vi "ExpFitHandle.vi"(8 "error in (no error)":errorcluster, 11 "Stand in":refnum<class "Stand.lvclass">) -> (0 "error out":errorcluster, 3 "Stand out":refnum<class "Stand.lvclass">)   [LabVIEW 2019, in "Stand.lvclass"]
uses:
  Stand.lvclass
  D:/GIT H4000/H4000/src/Device_class/Device.lvclass
  Stand.lvclass/Stand.ctl
  FPGA/TypeDef/DO index.ctl
  FPGA/TypeDef/AI index.ctl
  AI_class/AI.lvclass/AI.ctl
  AnalogComparator_class/AnalogComparator.lvclass/AnalogComparator.ctl
  OscillationClass/OscillationDetector.lvclass/OscillationDetector.ctl
  Device_class/Device.lvclass/Device.ctl
  249e4558-2c97-4a7e-83c2-ea0cef2754e0.vi
  AnalogComparator_class/GetStatus.vi
  OscillationClass/Read DATA.vi
  FPGA_API_class/FPGA API.lvclass
  ExpFitter/ExpFitter.lvclass
  Device_class/Device.lvclass
  AI_class/AI.lvclass
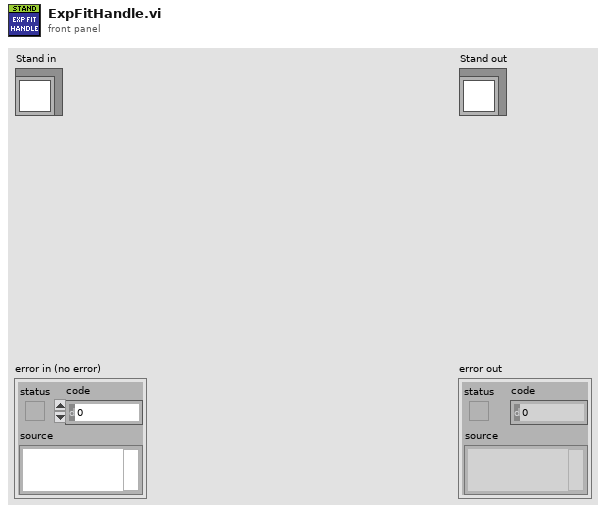
[diagram p1: front panel]
types:
  T1 = typedef "Step_Name.ctl" = enum16{"IDLE", "Filling", "Low Pressure", "Hi Pressure", "Abrupt Pressure Release", "Smooth Pressure Release", "Measuring Leakage Sensor 41.3", "Measuring Leakage Burette 42", "Alarm", "Stop Pump"}
  T2 = typedef "AI index.ctl" = u8
  T3 = typedef "DO index.ctl" = u8
  T4 = typedef "AI_Data.ctl" = cluster{"Stat Data":T5, "OutOfRangeMax":bool, "OutOfRangeMin":bool, "HIHI":bool, "HI":bool, "LO":bool, "LOLO":bool, "DATA N":T6, "DATA PERIOD":T6, "UPPER TH":dbl, "LOWER TH":dbl}
  T5 = typedef "AI Statistics Data.ctl" = cluster{"raw mean":dbl, "scl mean":dbl, "raw mean 1Hz":dbl, "scl mean 1Hz":dbl}
  T6 = typedef "DATA Oscill.ctl" = cluster{"SUM":dbl, "COUNTER":dbl, "MAX CURR":dbl, "MIN CURR":dbl, "AVR":dbl, "MAX":dbl, "MIN":dbl, "DELTA AVR":dbl, "DELTA MAX":dbl, "DELTA MIN":dbl, "PERIOD":dbl}
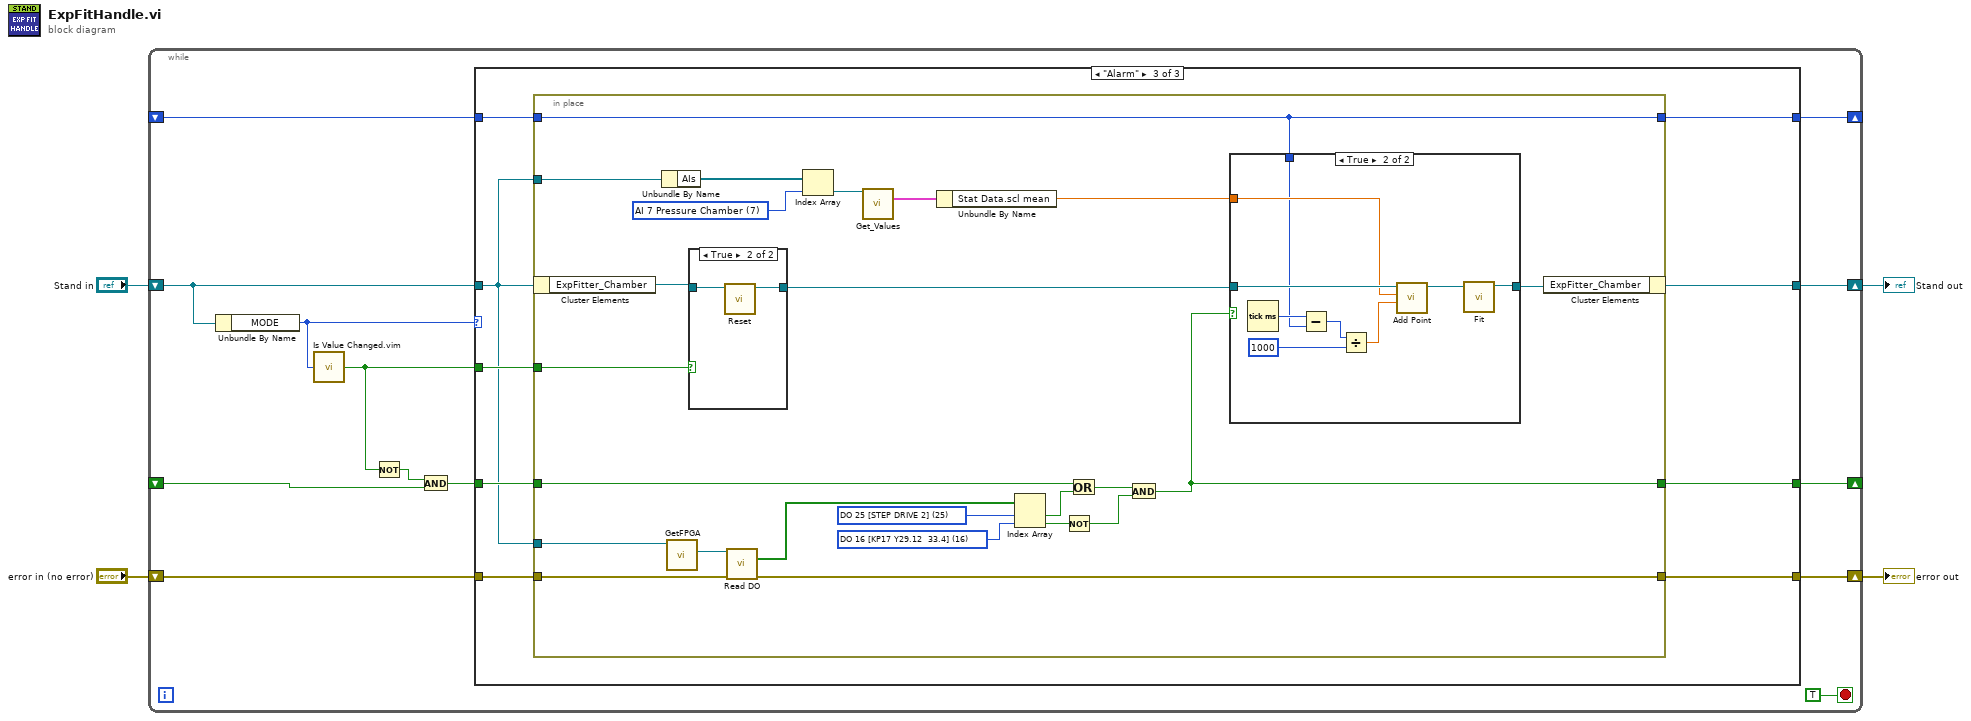
[diagram p0: block diagram]
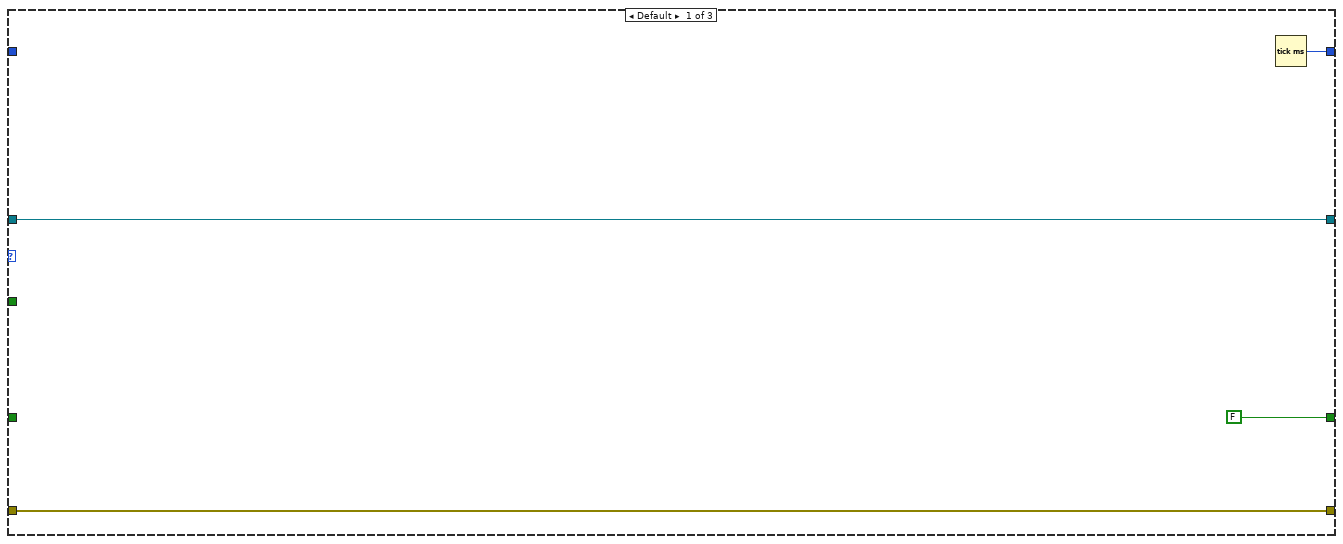
[diagram p2: hidden frame]
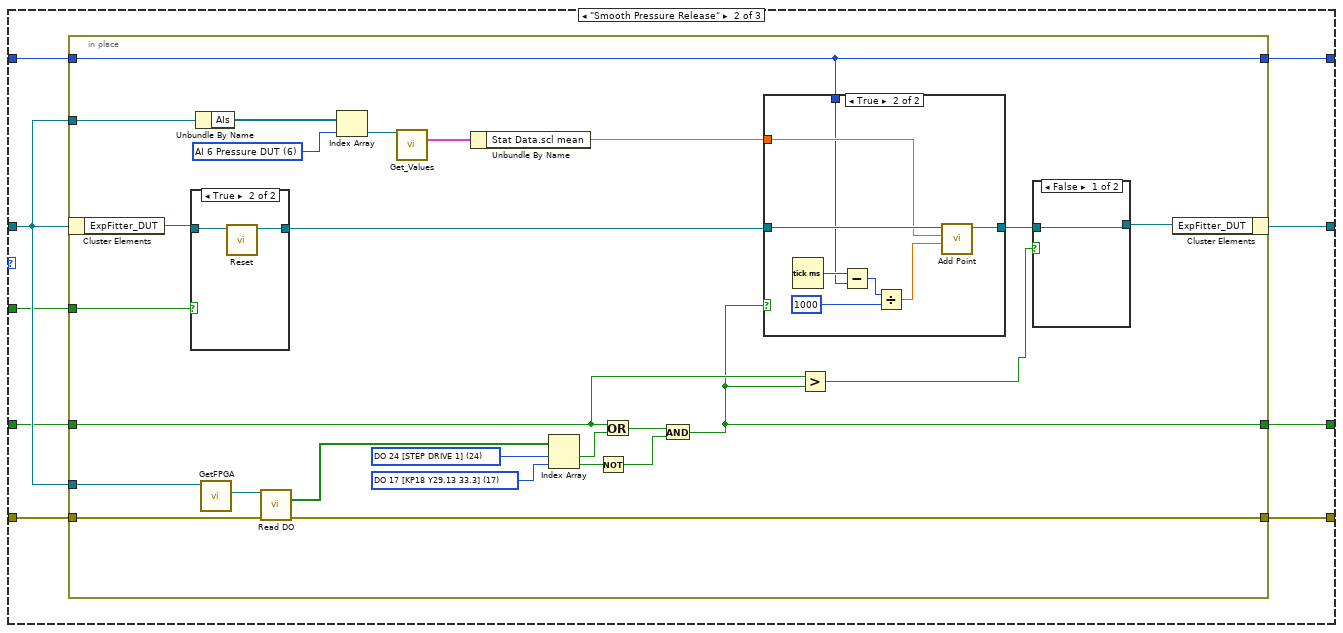
[diagram p3: hidden frame]
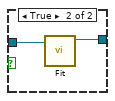
[diagram p4: hidden frame]
diagram:
  n1 = while {
    shift-right: [w15] -> w2
    shift-left: "error in (no error)" -> [w16]
    shift-right: [w17] -> w4
    shift-left: "Stand in" -> [w11]
    shift-right: [w12] -> _
    shift-left: _ -> [w8]
    shift-right: [w10] -> _
    shift-left: _ -> [w9]
    stop <- TRUE stop-if-true
    n2 = Unbundle By Name(w11) -> ("MODE"=w14:T1)
    n3 = call "Is Value Changed.vim"("value"=w14) -> ("changed or first call?"=w5:bool)
    n4 = Not(x=w5) -> (.not. x?=w6:bool)
    n5 = And(x=w6, y=w8) -> (x .and. y?=w7:bool)
    n6 = case shown="\"Alarm\"" w14 {
      tunnel: w11 -> [w21 w24 w72]
      tunnel: [w21 w25 w73] -> w17
      tunnel: w16 -> [w20 w30 w80]
      tunnel: [w20 w26 w74] -> w15
      tunnel: w5 -> [_ w23 w79]
      tunnel: [FALSE w29 w77] -> w12
      tunnel: w7 -> [_ w22 w78]
      tunnel: [w19 w28 w76] -> w10
      tunnel: w9 -> [_ w27 w75]
      frame Default {
        n7 = Tick Count (ms)() -> (millisecond timer value=w19:u32)
      }
      frame "Smooth Pressure Release" {
        n8 = in-place {
          in-place-border: w30 -> [w38]
          in-place-border: w23 -> [w55]
          in-place-border: w24 -> [w53]
          in-place-border: w22 -> [w33]
          in-place-border: [w32] -> w29
          in-place-border: [w39] -> w28
          in-place-border: w27 -> [w39]
          in-place-border: [w37] -> w26
          in-place-border: w24 -> [w36]
          w44 = T2 6 items=["AI 0 Cooling Station Level", "AI 1 Cooling Station Temp", "AI 2 Oil Supply Level", "AI 3 Oil Supply Temp", "AI 4 ", "AI 5 Pressure Haskel", "AI 6 Pressure DUT", "AI 7 Pressure Chamber", "AI 8 Pressure Air inlet", "AI 9 Pressure Air outlet", "AI 10 Pressure Messure Line"] ("AI index")
          w52 = T3 17 items=["DO 0 [KP1] [M12]", "DO 1 [ON KP2] [M21]", "DO 2 [ON KP3] [M24]", "DO 3 [WATER Y18.1 [DO3]]", "DO 4 [WATER Y18.2 [DO4]]", "DO 5 [KP6 Y29.1 33.7]", "DO 6 [KP7 Y29.2 33.8]", "DO 7 [KP8 Y29.3 33.9]", "DO 8 [KP9 Y29.4  33.12]", "DO 9 [KP10 Y29.5 33.1]", "DO 10 [KP11 Y29.6 33.2]", "DO 11 [KP12 Y29.7  33.13]", "DO 12 [KP13 Y29.8  33.11]", "DO 13 [KP14 Y29.9 33.10]", "DO 14 [KP15 Y29.10  33.6]", "DO 15 [KP16 Y29.11  33.5]", "DO 16 [KP17 Y29.12  33.4]", "DO 17 [KP18 Y29.13 33.3]", "DO 18 [AIR KP19]", "DO 19 [STEP DRIVE EN KP20]", "DO 20 [KP21 Y44.1 OPEN]", "DO 21 [ KP22 Y44.1 CLOSE]", "DO 22 [ KP23 Y44.2 OPEN]", "DO 23", "DO 24 [STEP DRIVE 1]", "DO 25 [STEP DRIVE 2]"] ("DO index")
          w51 = T3 24 items=["DO 0 [KP1] [M12]", "DO 1 [ON KP2] [M21]", "DO 2 [ON KP3] [M24]", "DO 3 [WATER Y18.1 [DO3]]", "DO 4 [WATER Y18.2 [DO4]]", "DO 5 [KP6 Y29.1 33.7]", "DO 6 [KP7 Y29.2 33.8]", "DO 7 [KP8 Y29.3 33.9]", "DO 8 [KP9 Y29.4  33.12]", "DO 9 [KP10 Y29.5 33.1]", "DO 10 [KP11 Y29.6 33.2]", "DO 11 [KP12 Y29.7  33.13]", "DO 12 [KP13 Y29.8  33.11]", "DO 13 [KP14 Y29.9 33.10]", "DO 14 [KP15 Y29.10  33.6]", "DO 15 [KP16 Y29.11  33.5]", "DO 16 [KP17 Y29.12  33.4]", "DO 17 [KP18 Y29.13 33.3]", "DO 18 [AIR KP19]", "DO 19 [STEP DRIVE EN KP20]", "DO 20 [KP21 Y44.1 OPEN]", "DO 21 [ KP22 Y44.1 CLOSE]", "DO 22 [ KP23 Y44.2 OPEN]", "DO 23", "DO 24 [STEP DRIVE 1]", "DO 25 [STEP DRIVE 2]"] ("DO index")
          n9 = in-place-cluster #1(w24) -> ("ExpFitter_DUT"=w56:refnum<class "ExpFitter.lvclass">)
          n10 = case shown="True" w55 {
            tunnel: w56 -> [w60 w62]
            tunnel: [w60 w61] -> w54
            frame False {
            }
            frame True {
              n11 = call "Reset.vi"("ExpFitter in"=w62) -> ("ExpFitter out"=w61:refnum<class "ExpFitter.lvclass">)  [unwired: 10 in]
            }
          }
          n12 = Unbundle By Name(w36) -> ("AIs"=w41:refnum<class "AI.lvclass">[])
          n13 = call "GetFPGA.vi"("Device in"=w53) -> ("FPGA API.lvclass"=w50:refnum<class "FPGA API.lvclass">)  [unwired: 10 in]
          n14 = call-dynamic "Read DO.vi"("FPGA API in"=w50, "error in (no error)"=w38) -> ("Ds"=w49:bool[], "error out"=w37:errorcluster)  [unwired: 11 in, 1 out]
          n15 = Index Array(array=w41, index=w44) -> (element=w42:refnum<class "AI.lvclass">)
          n16 = call "Get_Values.vi"("reference in"=w42) -> ("Data"=w43:T4)  [unwired: 14 in]
          n17 = Unbundle By Name(w43) -> ("Stat Data.scl mean"=w40:dbl)
          n18 = Index Array(array=w49, index #1=w51, index #2=w52) -> (element #1=w48:bool, element #2=w46:bool)
          n19 = Not(x=w46) -> (.not. x?=w45:bool)
          n20 = Or(x=w33, y=w48) -> (x .or. y?=w47:bool)
          n21 = And(x=w47, y=w45) -> (x .and. y?=w32:bool)
          n22 = case shown="True" w32 {
            tunnel: w54 -> [w63 w71]
            tunnel: [w63 w64] -> w35
            tunnel: w40 -> [_ w70]
            tunnel: w39 -> [_ w68]
            frame False {
            }
            frame True {
              n23 = Tick Count (ms)() -> (millisecond timer value=w69:u32)
              n24 = Subtract(x=w69, y=w68) -> (x-y=w67:u32)
              n25 = Divide(x=w67, y=u32 1000) -> (x/y=w65:dbl)
              n26 = call "Add Point.vi"("X"=w65, "Y"=w70, "ExpFitter in"=w71) -> ("ExpFitter out"=w64:refnum<class "ExpFitter.lvclass">)  [unwired: 8 in]
            }
          }
          n27 = Greater?(x=w33, y=w32) -> (0:w31:bool)
          n28 = case shown="False" w31 {
            tunnel: w35 -> [w57 w59]
            tunnel: [w57 w58] -> w34
            frame False {
            }
            frame True {
              n29 = call "Fit.vi"("ExpFitter in"=w59) -> ("ExpFitter out"=w58:refnum<class "ExpFitter.lvclass">)  [unwired: 10 in]
            }
          }
          n30 = in-place-cluster #1("ExpFitter_DUT"=w34) -> (w25:refnum<class "Stand.lvclass">)
        }
      }
      frame "Alarm" {
        n31 = in-place {
          in-place-border: w80 -> [w83]
          in-place-border: w79 -> [w103]
          in-place-border: w72 -> [w101]
          in-place-border: w78 -> [w96]
          in-place-border: [w91] -> w77
          in-place-border: [w84] -> w76
          in-place-border: w75 -> [w84]
          in-place-border: [w82] -> w74
          in-place-border: w72 -> [w81]
          w89 = T2 7 items=["AI 0 Cooling Station Level", "AI 1 Cooling Station Temp", "AI 2 Oil Supply Level", "AI 3 Oil Supply Temp", "AI 4 ", "AI 5 Pressure Haskel", "AI 6 Pressure DUT", "AI 7 Pressure Chamber", "AI 8 Pressure Air inlet", "AI 9 Pressure Air outlet", "AI 10 Pressure Messure Line"] ("AI index")
          w100 = T3 16 items=["DO 0 [KP1] [M12]", "DO 1 [ON KP2] [M21]", "DO 2 [ON KP3] [M24]", "DO 3 [WATER Y18.1 [DO3]]", "DO 4 [WATER Y18.2 [DO4]]", "DO 5 [KP6 Y29.1 33.7]", "DO 6 [KP7 Y29.2 33.8]", "DO 7 [KP8 Y29.3 33.9]", "DO 8 [KP9 Y29.4  33.12]", "DO 9 [KP10 Y29.5 33.1]", "DO 10 [KP11 Y29.6 33.2]", "DO 11 [KP12 Y29.7  33.13]", "DO 12 [KP13 Y29.8  33.11]", "DO 13 [KP14 Y29.9 33.10]", "DO 14 [KP15 Y29.10  33.6]", "DO 15 [KP16 Y29.11  33.5]", "DO 16 [KP17 Y29.12  33.4]", "DO 17 [KP18 Y29.13 33.3]", "DO 18 [AIR KP19]", "DO 19 [STEP DRIVE EN KP20]", "DO 20 [KP21 Y44.1 OPEN]", "DO 21 [ KP22 Y44.1 CLOSE]", "DO 22 [ KP23 Y44.2 OPEN]", "DO 23", "DO 24 [STEP DRIVE 1]", "DO 25 [STEP DRIVE 2]"] ("DO index")
          w99 = T3 25 items=["DO 0 [KP1] [M12]", "DO 1 [ON KP2] [M21]", "DO 2 [ON KP3] [M24]", "DO 3 [WATER Y18.1 [DO3]]", "DO 4 [WATER Y18.2 [DO4]]", "DO 5 [KP6 Y29.1 33.7]", "DO 6 [KP7 Y29.2 33.8]", "DO 7 [KP8 Y29.3 33.9]", "DO 8 [KP9 Y29.4  33.12]", "DO 9 [KP10 Y29.5 33.1]", "DO 10 [KP11 Y29.6 33.2]", "DO 11 [KP12 Y29.7  33.13]", "DO 12 [KP13 Y29.8  33.11]", "DO 13 [KP14 Y29.9 33.10]", "DO 14 [KP15 Y29.10  33.6]", "DO 15 [KP16 Y29.11  33.5]", "DO 16 [KP17 Y29.12  33.4]", "DO 17 [KP18 Y29.13 33.3]", "DO 18 [AIR KP19]", "DO 19 [STEP DRIVE EN KP20]", "DO 20 [KP21 Y44.1 OPEN]", "DO 21 [ KP22 Y44.1 CLOSE]", "DO 22 [ KP23 Y44.2 OPEN]", "DO 23", "DO 24 [STEP DRIVE 1]", "DO 25 [STEP DRIVE 2]"] ("DO index")
          n32 = in-place-cluster #2(w72) -> ("ExpFitter_Chamber"=w104:refnum<class "ExpFitter.lvclass">)
          n33 = Unbundle By Name(w81) -> ("AIs"=w86:refnum<class "AI.lvclass">[])
          n34 = call "GetFPGA.vi"("Device in"=w101) -> ("FPGA API.lvclass"=w98:refnum<class "FPGA API.lvclass">)  [unwired: 10 in]
          n35 = case shown="True" w103 {
            tunnel: w104 -> [w105 w107]
            tunnel: [w105 w106] -> w102
            frame False {
            }
            frame True {
              n36 = call "Reset.vi"("ExpFitter in"=w107) -> ("ExpFitter out"=w106:refnum<class "ExpFitter.lvclass">)  [unwired: 10 in]
            }
          }
          n37 = call-dynamic "Read DO.vi"("FPGA API in"=w98, "error in (no error)"=w83) -> ("Ds"=w97:bool[], "error out"=w82:errorcluster)  [unwired: 11 in, 1 out]
          n38 = Index Array(array=w86, index=w89) -> (element=w87:refnum<class "AI.lvclass">)
          n39 = call "Get_Values.vi"("reference in"=w87) -> ("Data"=w88:T4)  [unwired: 14 in]
          n40 = Unbundle By Name(w88) -> ("Stat Data.scl mean"=w85:dbl)
          n41 = Index Array(array=w97, index #1=w99, index #2=w100) -> (element #1=w95:bool, element #2=w93:bool)
          n42 = Not(x=w93) -> (.not. x?=w92:bool)
          n43 = Or(x=w96, y=w95) -> (x .or. y?=w94:bool)
          n44 = And(x=w94, y=w92) -> (x .and. y?=w91:bool)
          n45 = case shown="True" w91 {
            tunnel: w102 -> [w108 w117]
            tunnel: [w108 w109] -> w90
            tunnel: w85 -> [_ w116]
            tunnel: w84 -> [_ w114]
            frame False {
            }
            frame True {
              n46 = Tick Count (ms)() -> (millisecond timer value=w115:u32)
              n47 = Subtract(x=w115, y=w114) -> (x-y=w113:u32)
              n48 = Divide(x=w113, y=u32 1000) -> (x/y=w111:dbl)
              n49 = call "Add Point.vi"("X"=w111, "Y"=w116, "ExpFitter in"=w117) -> ("ExpFitter out"=w110:refnum<class "ExpFitter.lvclass">)  [unwired: 8 in]
              n50 = call "Fit.vi"("ExpFitter in"=w110) -> ("ExpFitter out"=w109:refnum<class "ExpFitter.lvclass">)  [unwired: 10 in]
            }
          }
          n51 = in-place-cluster #2("ExpFitter_Chamber"=w90) -> (w73:refnum<class "Stand.lvclass">)
        }
      }
    }
  }
  "error out" <- w2
  "Stand out" <- w4
